vi "Update Active Attribute Value.vi"(8 "error in (no error)":errorcluster, 10 "Data":variant, 11 "Test Step Dialog in":refnum<class "Test Step Dialog.lvclass">) -> (0 "error out":errorcluster, 3 "Test Step Dialog out":refnum<class "Test Step Dialog.lvclass">)   [LabVIEW 2017, in "Test Step Dialog.lvclass"]
uses:
  Test Step Dialog.lvclass
  Test Step Dialog.lvclass/Test Step Dialog.ctl
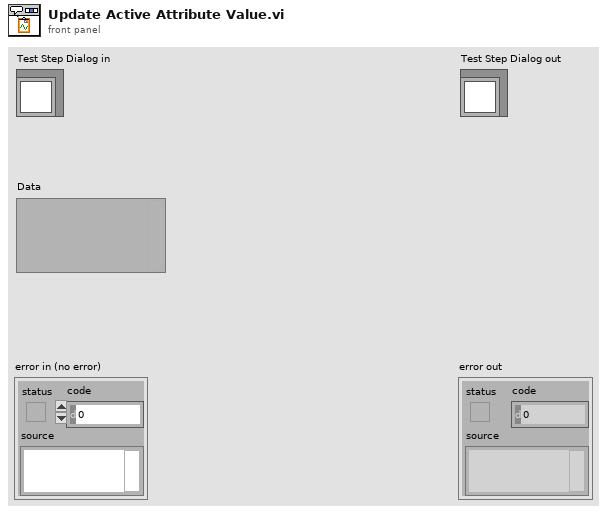
[diagram p1: front panel]
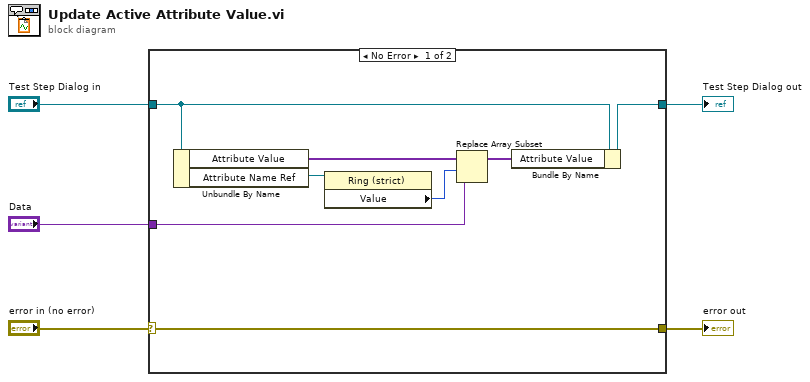
[diagram p0: block diagram]
diagram:
  n1 = case shown="No Error" "error in (no error)" {
    selector: "error in (no error)" -> [w13 w14]
    tunnel: [w7 w15] -> w5
    tunnel: "Test Step Dialog in" -> [w8 w15]
    tunnel: [w13 w14] -> w2
    tunnel: "Data" -> [w9 _]
    frame No Error {
      n2 = Unbundle By Name(w8) -> ("Attribute Value"=w11:variant[], "Attribute Name Ref"=w12:refnum<vi>)
      n3 = property class="Ring (strict)"(reference=w12) -> ("Value"=w10:u16)  [unwired: 1 in, 2 out]
      n4 = Replace Array Subset(array=w11, new element=w9, index=w10) -> (w6:variant[])
      n5 = Bundle By Name(cluster=w8, "Attribute Value"=w6) -> (w7:refnum<class "Test Step Dialog.lvclass">)
    }
    frame Error {
    }
  }
  "error out" <- w2
  "Test Step Dialog out" <- w5
